vi "MALT XmlNodeReadValue Int.vi"(8 "error in":errorcluster, 10 "XPath":string, 11 "XML File Path":path) -> (0 "error out":errorcluster, 3 "number":i32)   [LabVIEW 2018, in "AltonTech MALT200817.lvlib"]
uses:
  AltonTech MALT200817.lvlib
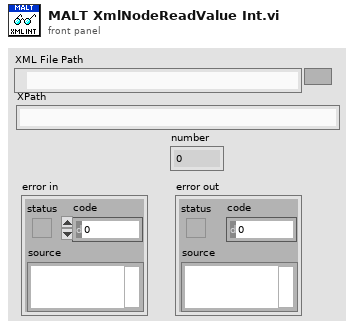
[diagram p1: front panel]
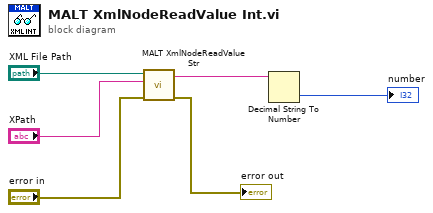
[diagram p0: block diagram]
diagram:
  n1 = call "MALT XmlNodeReadValue Str.vi"("error in"="error in", "XPath"="XPath", "XML File Path"="XML File Path") -> ("error out"=→"error out":errorcluster, "value"=w3:string)  [unwired: 7 in]
  n2 = Decimal String To Number(string=w3) -> (number=→"number":i32)  [unwired: 2 in, 1 out]
